vi "Basic_vi_Recursively search folders for file.vi"(1 "File name":string="result", 7 "Folder Path":path caption="Root path") -> (8 "All folders containing .txt and .bin files":path[](array[path]))   [LabVIEW 2020, in "BasicVIs.lvlib"]
uses:
  BasicVIs.lvlib
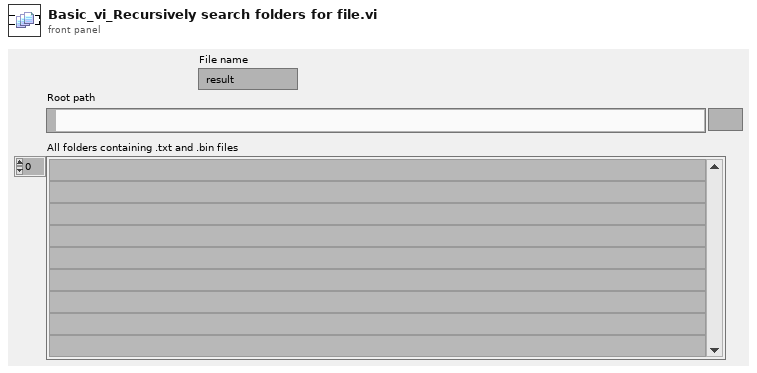
[diagram p1: front panel]
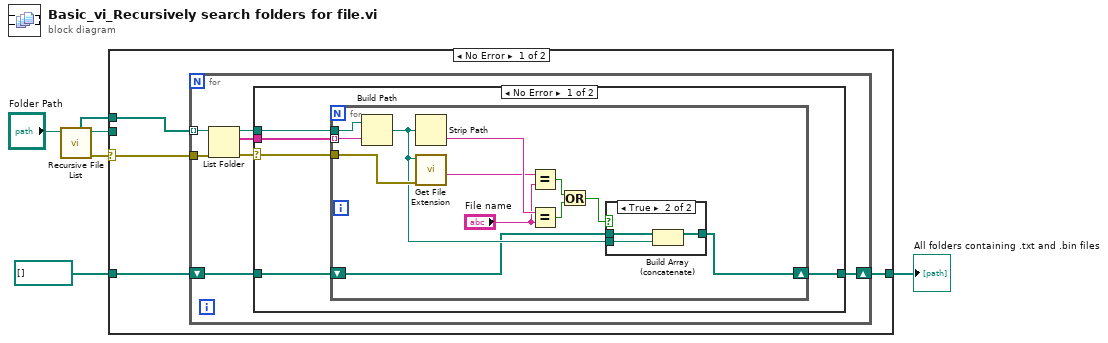
[diagram p0: block diagram]
diagram:
  n1 = call <vilib>:"Recursive File List.vi"("Folder Path"="Folder Path") -> ("error out"=w5:errorcluster, "dup Folder Path"=w2:path, "All Folders"=w4:path[])  [unwired: 6 in, 2 out]
  n2 = case shown="No Error" w5 {
    selector: w5 -> [w9 _]
    tunnel: w4 -> [w10 _]
    tunnel: [w8 w40] -> w1
    tunnel: path[] [] -> [w7 w40]
    tunnel: w2 -> [_ _]
    frame No Error {
      n3 = for {
        tunnel: w10 -> [w17] mode=indexing
        tunnel: w9 -> [w13]
        shift-right: [w11] -> w8
        shift-left: w7 -> [w12]
        n4 = List Folder(path=w17, error in=w13) -> (path out=w16:path, filenames=w15:string[], error out=w14:errorcluster)  [unwired: 2 in, 1 out]
        n5 = case shown="No Error" w14 {
          selector: w14 -> [w21 _]
          tunnel: w16 -> [w20 _]
          tunnel: w15 -> [w22 _]
          tunnel: w12 -> [w19 w39]
          tunnel: [w18 w39] -> w11
          frame No Error {
            n6 = for {
              tunnel: w20 -> [w34]
              tunnel: w22 -> [w33] mode=indexing
              tunnel: w21 -> [w31]
              shift-right: [w23] -> w18
              shift-left: w19 -> [w24]
              n7 = Build Path(base path=w34, name or relative path=w33) -> (appended path=w25:path)
              n8 = Strip Path(path=w25) -> (name=w32:string)  [unwired: 1 out]
              n9 = call <vilib>:"Get File Extension.vi"("error in (no error)"=w31, "file"=w25) -> ("filename without extension"=w30:string)  [unwired: 5 in, 4 out]
              n10 = Equal?(x=w30, y="File name") -> (x = y?=w27:bool)
              n11 = Equal?(x=w32, y="File name") -> (x = y?=w28:bool)
              n12 = Or(x=w27, y=w28) -> (x .or. y?=w26:bool)
              n13 = case shown="True" w26 {
                tunnel: [w35 w38] -> w23
                tunnel: w25 -> [_ w37]
                tunnel: w24 -> [w35 w36]
                frame False {
                }
                frame True {
                  n14 = Build Array (concatenate)(w36, w37) -> (w38:path[])
                }
              }
            }
          }
          frame Error {
          }
        }
      }
    }
    frame Error {
    }
  }
  "All folders containing .txt and .bin files" <- w1
